vi "Multiply via Server 2.vi"(1 "Unique 8b identifier":u8, 4 "Input B":fxp<+/-,18,1>, 5 "Input A":fxp<+/-,18,1>) -> (0 "Output":fxp<+/-,18,1>)   [LabVIEW 2009]
doc: "Major note from gray:\nThere is a possibility that this vi will frack your shit. It is designed to be non re-entrant (clone copy), and it is also designed to support 2^8 clients, each client basically using the multiplication server periodically (and maintaining a unique 8b identifier). IF the server is monopolized by one client, this client may get screwed up by an identical looking but much older packet. The client's clone of this vi will maintain an 8 bit register to indicate a count but only 6 bits are read! 2^6 is 64 so, given the 69 memory locations the vi might be reading, there is a chance that it will read an incorect value (the 64th oldest one) from those five insecure locations. The timing of this vi is designed to maximize the chance that the first newest number is read, but it is possible that the channel watcher vi will execute before the value is added, and in this case the channel watcher will search through all 69 locations before searching the most likely one again. If this happens the watcher will notice this older datapoint in one of these 5 insecure locations and will use it instead of the new multiplication. \nThe solution to this problem is to avoid monopolizing channels and in the worst case divide the multiplication from one client between two clones."
uses:
  Motor Control Global.vi
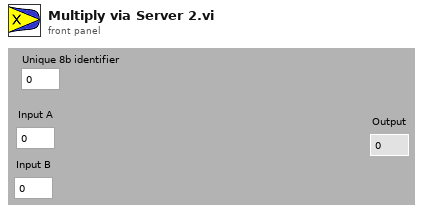
[diagram p1: front panel]
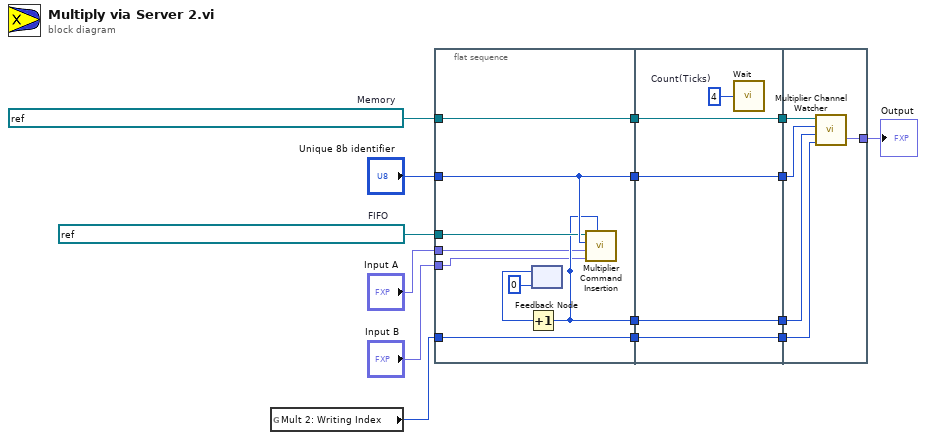
[diagram p0: block diagram]
diagram:
  w2 = refnum<k21> "Multiplier 2 FIFO In : [8b Identifier; 20b args; 18b fxp; 18b fxp]"  # FIFO
  w3 = refnum<k21> "Multiplier 2 Block Memory Out: [8b Identifier; 6b args; 18b fxp output]"  # Memory
  n1 = global read "Motor Control Global.vi" "Mult 2: Writing Index"() -> (w1:u32)
  n2 = flat-sequence {
    tunnel: [w24] -> w11
    tunnel: [w23] -> w10
    tunnel: [w19] -> w9
    tunnel: [w20] -> w8
    tunnel: "Unique 8b identifier" -> [w24]
    tunnel: w2 -> [w22]
    tunnel: w3 -> [w23]
    tunnel: w1 -> [w19]
    tunnel: "Input A" -> [w17]
    tunnel: "Input B" -> [w16]
    tunnel: w11 -> [w29]
    tunnel: [w29] -> w7
    tunnel: w10 -> [w28]
    tunnel: [w28] -> w6
    tunnel: w9 -> [w27]
    tunnel: [w27] -> w5
    tunnel: w8 -> [w26]
    tunnel: [w26] -> w4
    tunnel: w7 -> [w34]
    tunnel: w6 -> [w33]
    tunnel: w5 -> [w32]
    tunnel: w4 -> [w31]
    tunnel: [w30] -> w13
    frame #0 {
      n3 = feedback #1(u8 0) -> (w21:u8)
      n4 = Increment(x=w21) -> (x+1=w20:u8)
      n5 = call "Multiplier Command Insertion.vi"("Counter Descriminator"=w20, "Input B"=w16, "Input A"=w17, "Channel Identifier"=w24, "FIFO"=w22) -> ()  [unwired: 6 in, 1 out]
    }
    frame #1 {
      w25 = u32 4  # Count(Ticks)
      n6 = call "Wait"("Count(Ticks)"=w25) -> ()  [unwired: 1 out]
    }
    frame #2 {
      n7 = call "Multiplier Channel Watcher.vi"("Writing Index Start"=w32, "Count to match"=w31, "Watched Channel"=w34, "Block Memory"=w33) -> ("Multiplication Result"=w30:fxp<+/-,18,1>)  [unwired: 1 out]
    }
  }
  "Output" <- w13
